vi "Chart.vi"(0 "PictureIn":picture, 5 "x":i16=11, 7 "y":i16=50, 9 "colorRectangle":u32(colorbox)=16860, 11 "error in (no error)":errorcluster) -> (4 "ChartOut":picture, 15 "error out":errorcluster)   [LabVIEW 2014]
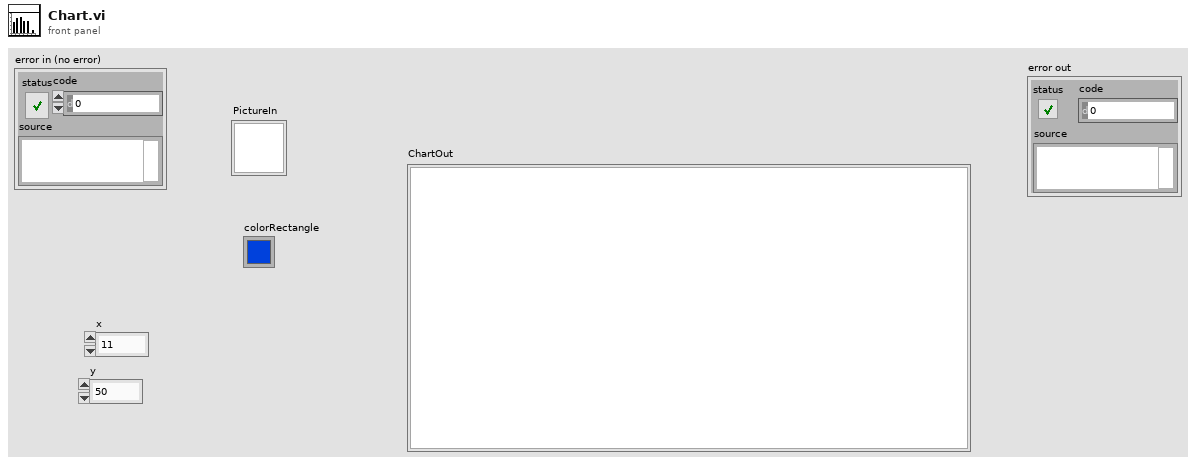
[diagram p1: front panel]
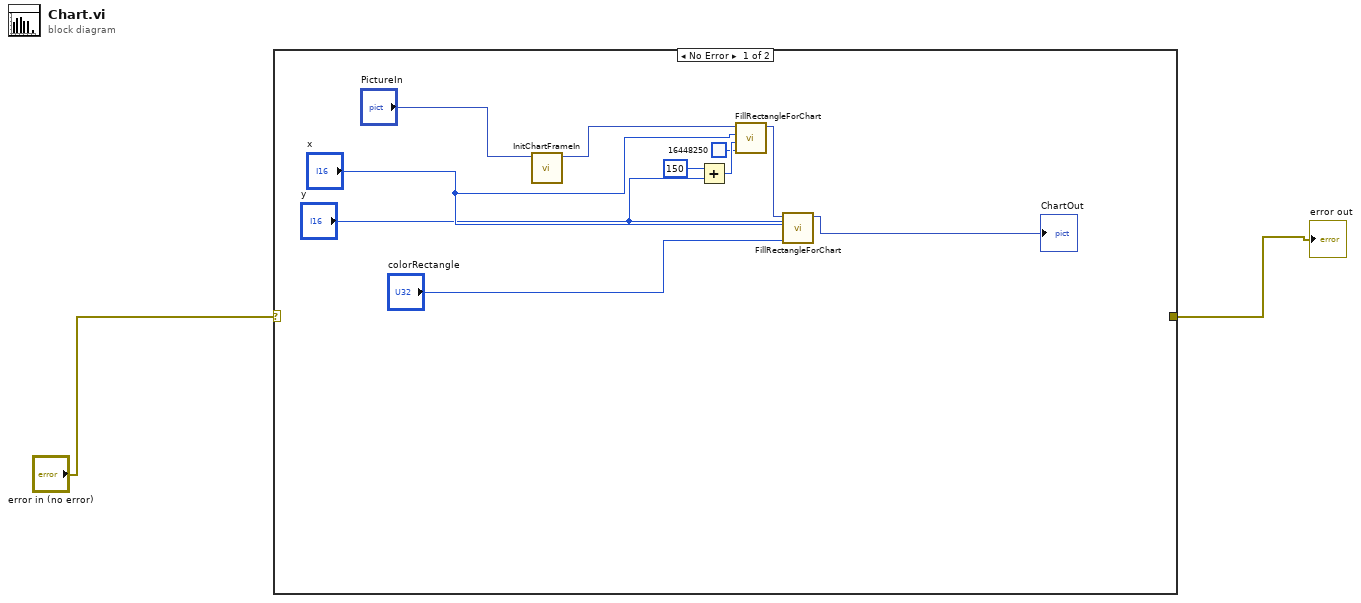
[diagram p0: block diagram]
diagram:
  n1 = case shown="No Error" "error in (no error)" {
    selector: "error in (no error)" -> [_ w13]
    tunnel: [_ w13] -> w1
    frame No Error {
      n2 = call "InitChartFrameIn.vi"("PictureIn"="PictureIn") -> ("PictureOut"=w9:picture)  [unwired: 10 in]
      n3 = Add(x=i16 150, y="y") -> (x+y=w4:i16)
      n4 = call "FillRectangleForChart.vi"("colorRectangle"=u32 16448250, "y"=w4, "x"="x", "PictureIn"=w9) -> ("PictureOut"=w8:picture)  [unwired: 7 in]
      n5 = call "FillRectangleForChart.vi"("colorRectangle"="colorRectangle", "y"="y", "x"="x", "PictureIn"=w8) -> ("PictureOut"=→"ChartOut":picture)  [unwired: 7 in]
    }
    frame Error {
    }
  }
  "error out" <- w1
